vi "DataLog Pull DB.vi"(5 "LuaVIEW reference in":T2, 11 "error in (no error)":errorcluster) -> (4 "database info":T1, 6 "LuaVIEW reference out":T2, 15 "error out":errorcluster)   [LabVIEW 2012]
doc: "Helper function for DB methods and other tag log functions. Pulls a DB object from the stack and casts the reference."
uses:
  typedefs/t_DataLog Database Info Pane.ctl
  luaview/typedefs/t_LuaVIEW Reference.ctl
  luaview/subvis/private/LuaVIEW Pull (object).vi
panel:
  in  "Case Constant\n(See Context Help)":bool=TRUE
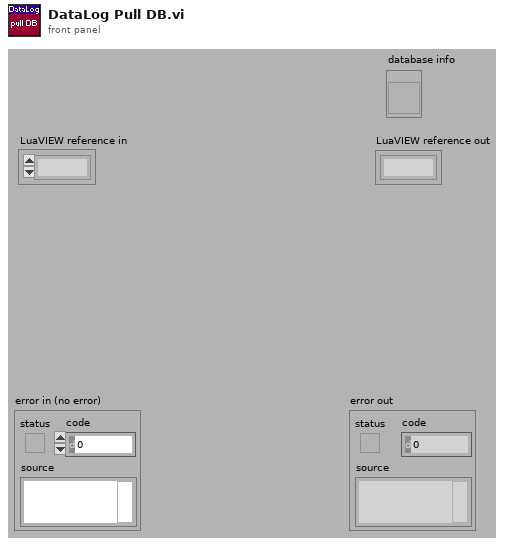
[diagram p1: front panel]
types:
  T1 = typedef "t_DataLog Database Info Pane.ctl" = refnum<vi>
  T2 = typedef "t_LuaVIEW Reference.ctl" = refnum<k1>
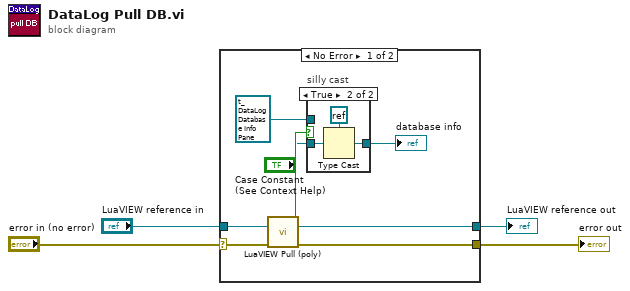
[diagram p0: block diagram]
diagram:
  n1 = case shown="No Error" "error in (no error)" {
    selector: "error in (no error)" -> [w12 w18]
    tunnel: [w5 w18] -> w4
    tunnel: "LuaVIEW reference in" -> [w11 w17]
    tunnel: [w6 w17] -> w1
    frame No Error {
      n2 = call-poly "LuaVIEW Pull (poly).vi"("LuaVIEW reference in"=w11, "error in (no error)"=w12) -> ("object refnum"=w9:refnum<vi>, "LuaVIEW reference out"=w6:T2, "error out"=w5:errorcluster)  [unwired: 10 in, 1 out]
      n3 = case "silly cast" shown="True" "Case Constant\n(See Context Help)" {
        tunnel: T1 refnum ("database info in (pull object)") -> [w13 _]
        tunnel: w9 -> [_ w14]
        tunnel: [w13 w16] -> w7
        frame False {
        }
        frame True {
          n4 = Type Cast(type=refnum<k0> refnum, x=w14) -> (*(type *) &x=w16:refnum<k0>)
        }
      }
      "database info" <- w7
    }
    frame Error {
    }
  }
  "error out" <- w4
  "LuaVIEW reference out" <- w1
